vi "New WebSocket Client.vi"(5 "Realm":string, 7 "Address":string, 11 "error in (no error)":errorcluster) -> (4 "reference out":refnum<class "WAMP Client.lvclass">, 15 "error out":errorcluster)   [LabVIEW 2020, in "wamplv.lvlib" / "WAMP Client.lvclass"]
uses:
  WAMP Client.lvclass
  Comm Handlers/Websocket Handler/Websocket Handler.lvclass
  C:/wamplv/Comm Handlers/ICommHandler/ICommHandler.lvclass
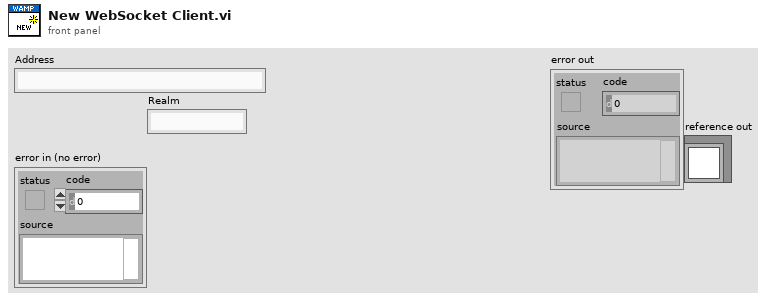
[diagram p1: front panel]
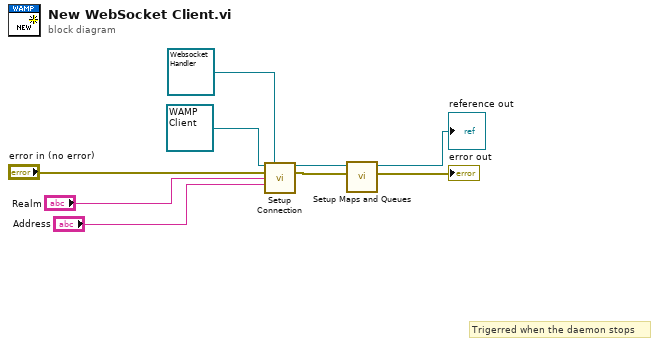
[diagram p0: block diagram]
diagram:
  # "Trigerred when the daemon stops"
  n1 = call-dynamic "Setup Connection.vi"("WAMP Client in"=refnum<class "WAMP Client.lvclass"> refnum ("WAMP Client.lvclass"), "ICommHandler.lvclass"=refnum<class "Websocket Handler.lvclass"> refnum ("Websocket Handler.lvclass"), "error in (no error)"="error in (no error)", "Realm"="Realm", "Address"="Address") -> ("WAMP Client out"=w4:refnum<class "WAMP Client.lvclass">, "error out"=w3:errorcluster)  [unwired: 9 in]
  n2 = call-dynamic "Setup Maps and Queues.vi"("error in (no error)"=w3, "WAMP Client in"=w4) -> ("error out"=→"error out":errorcluster, "WAMP Client out"=→"reference out":refnum<class "WAMP Client.lvclass">)  [unwired: 8 in]
